vi "Handler - Set Testing State.vi"(8 "error in":errorcluster, 10 "Data In":bool, 11 "File IO Data in":T1={"Work Order Folder"=path "", "Runcount File"=path "", "Report Template Folder"=path "", "Report Folder"=path "", "Report File"=path "", "APU Setup Folder"=path "", "Testing State"=FALSE, "Recording State"=FALSE, "TDMS File Ref"=refnum, "APU Setup File Ref"=refnum, "APU Select"="<Select>", "Test Information"={"APU Part Number:"="", "Model:"="", "Serial Number:"="", "Customer:"="", "Work Order:"="", "Repair Level:"="", "Pre or Post SB"=""}, "Crash Log Data"=[], "Group Name"="", "APU Setup File"={"Sensor Info"=[], "Calibration Info"=[], "CMM Table 106"=[], "CMM Table 106B "=[], "Accel Config"=[], "Report Sheet 1"=[], "Report Sheet 2"=[], "Report Sheet 3"=[]}, "APURunCount"=0}) -> (0 "error out":errorcluster, 3 "File IO Data out":T1={"Work Order Folder"=path "", "Runcount File"=path "", "Report Template Folder"=path "", "Report Folder"=path "", "Report File"=path "", "APU Setup Folder"=path "", "Testing State"=FALSE, "Recording State"=FALSE, "TDMS File Ref"=refnum, "APU Setup File Ref"=refnum, "APU Select"="<Select>", "Test Information"={"APU Part Number:"="", "Model:"="", "Serial Number:"="", "Customer:"="", "Work Order:"="", "Repair Level:"="", "Pre or Post SB"=""}, "Crash Log Data"=[], "Group Name"="", "APU Setup File"={"Sensor Info"=[], "Calibration Info"=[], "CMM Table 106"=[], "CMM Table 106B "=[], "Accel Config"=[], "Report Sheet 1"=[], "Report Sheet 2"=[], "Report Sheet 3"=[]}, "APURunCount"=0})   [LabVIEW 2018]
doc: "Handle events that occur when the testing state changes. Includes the initialization of the TMDS file."
uses:
  Top Level/Shared Controls/Acq Data.ctl
  Top Level/Shared Controls/Calculated Data.ctl
  Top Level/Shared Controls/All Data Cluster.ctl
  Top Level/Shared Controls/Analyzed Data Sets.ctl
  Controller (Host)/Public Controls/Test Information.ctl
  Controller (Host)/Controller (Host).lvlib
  Private Controls/File IO Data.ctl
  File IO.lvlib
  Controller (Host)/Public Controls/APU Select.ctl
  Top Level/Shared Controls/APU Setup File.ctl
panel:
  # "Test Information:"
  # "Test Information:"
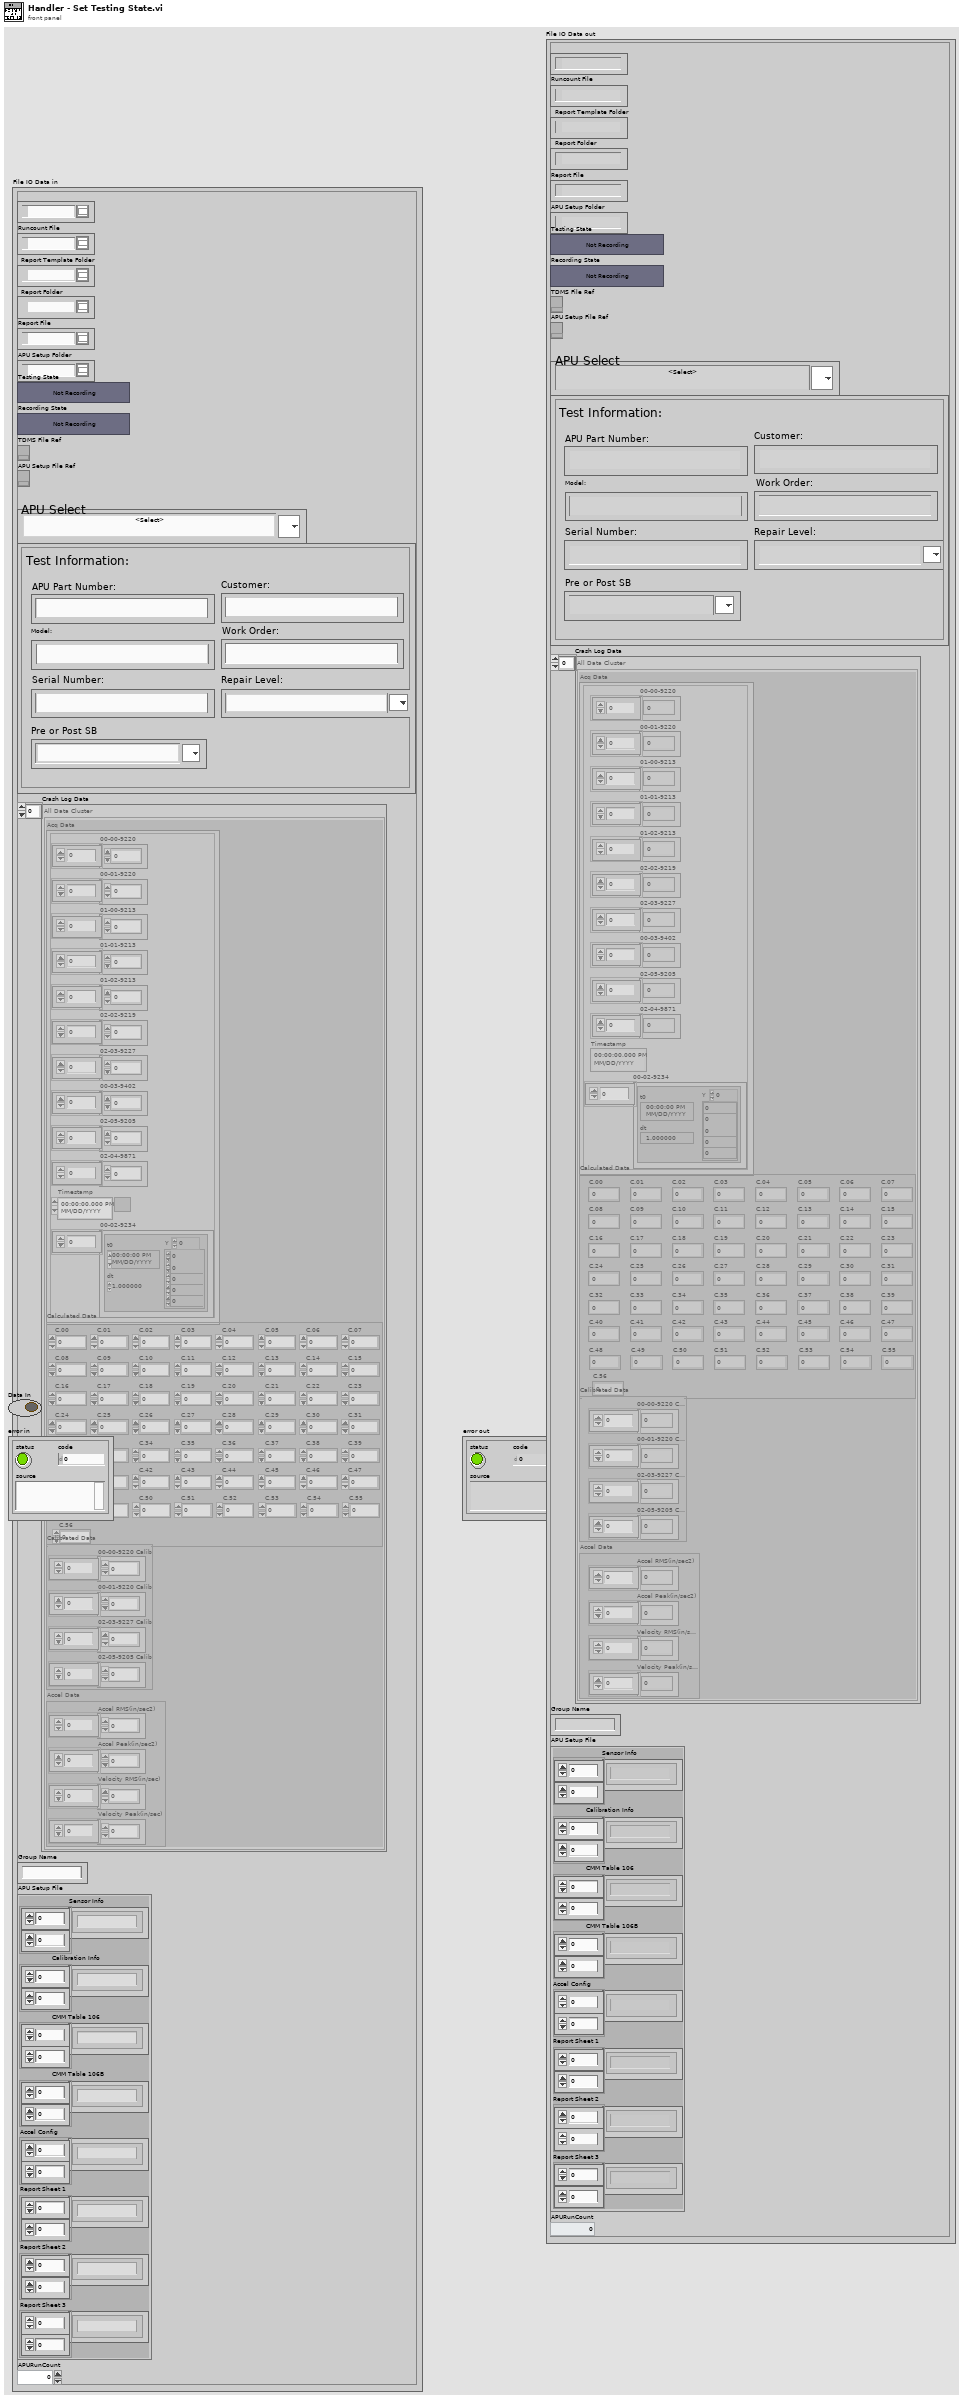
[diagram p1: front panel]
types:
  T1 = typedef "File IO.lvlib/File IO Data.ctl" = cluster{"Work Order Folder":path, "Runcount File":path, "Report Template Folder":path, "Report Folder":path, "Report File":path, "APU Setup Folder":path, "Testing State":bool, "Recording State":bool, "TDMS File Ref":refnum<k34>, "APU Setup File Ref":refnum<k34>, "APU Select":T2, "Test Information":T3, "Crash Log Data":T4, "Group Name":string, "APU Setup File":T8, "APURunCount":u32}
  T2 = typedef "Controller (Host).lvlib/APU Select.ctl" = string
  T3 = typedef "Controller (Host).lvlib/Test Information.ctl" = cluster{"APU Part Number:":string, "Model:":string, "Serial Number:":string, "Customer:":string, "Work Order:":string, "Repair Level:":string, "Pre or Post SB":string}
  T4 = typedef "Analyzed Data Sets.ctl" = T5[]
  T5 = typedef "All Data Cluster.ctl" = cluster{"Acq Data":T6, "Calculated Data":T7, "Calibrated Data":cluster{"00-00-9220 Calib":dbl[], "00-01-9220 Calib":dbl[], "02-03-9227 Calib":dbl[], "02-05-9205 Calib":dbl[]}, "Accel Data":cluster{"Accel RMS(in/sec2)":dbl[], "Accel Peak(in/sec2)":dbl[], "Velocity RMS(in/sec)":dbl[], "Velocity Peak(in/sec)":dbl[]}}
  T6 = typedef "Acq Data.ctl" = cluster{"00-00-9220":dbl[], "00-01-9220":dbl[], "01-00-9213":dbl[], "01-01-9213":dbl[], "01-02-9213":dbl[], "02-02-9219":dbl[], "02-03-9227":dbl[], "00-03-9402":dbl[], "02-05-9205":dbl[], "02-04-9871":dbl[], "Timestamp":timestamp, "00-02-9234":waveform(sgl)[]}
  T7 = typedef "Calculated Data.ctl" = cluster{"C.00":dbl, "C.01":dbl, "C.02":dbl, "C.03":dbl, "C.04":dbl, "C.05":dbl, "C.06":dbl, "C.07":dbl, "C.08":dbl, "C.09":dbl, "C.10":dbl, "C.11":dbl, "C.12":dbl, "C.13":dbl, "C.14":dbl, "C.15":dbl, "C.16":dbl, "C.17":dbl, "C.18":dbl, "C.19":dbl, "C.20":dbl, "C.21":dbl, "C.22":dbl, "C.23":dbl, "C.24":dbl, "C.25":dbl, "C.26":dbl, "C.27":dbl, "C.28":dbl, "C.29":dbl, "C.30":dbl, "C.31":dbl, "C.32":dbl, "C.33":dbl, "C.34":dbl, "C.35":dbl, "C.36":dbl, "C.37":dbl, "C.38":dbl, "C.39":dbl, "C.40":dbl, "C.41":dbl, "C.42":dbl, "C.43":dbl, "C.44":dbl, "C.45":dbl, "C.46":dbl, "C.47":dbl, "C.48":dbl, "C.49":dbl, "C.50":dbl, "C.51":dbl, "C.52":dbl, "C.53":dbl, "C.54":dbl, "C.55":dbl, "C.56":dbl}
  T8 = typedef "APU Setup File.ctl" = cluster{"Sensor Info":string[][], "Calibration Info":string[][], "CMM Table 106":string[][], "CMM Table 106B ":string[][], "Accel Config":string[][], "Report Sheet 1":string[][], "Report Sheet 2":string[][], "Report Sheet 3":string[][]}
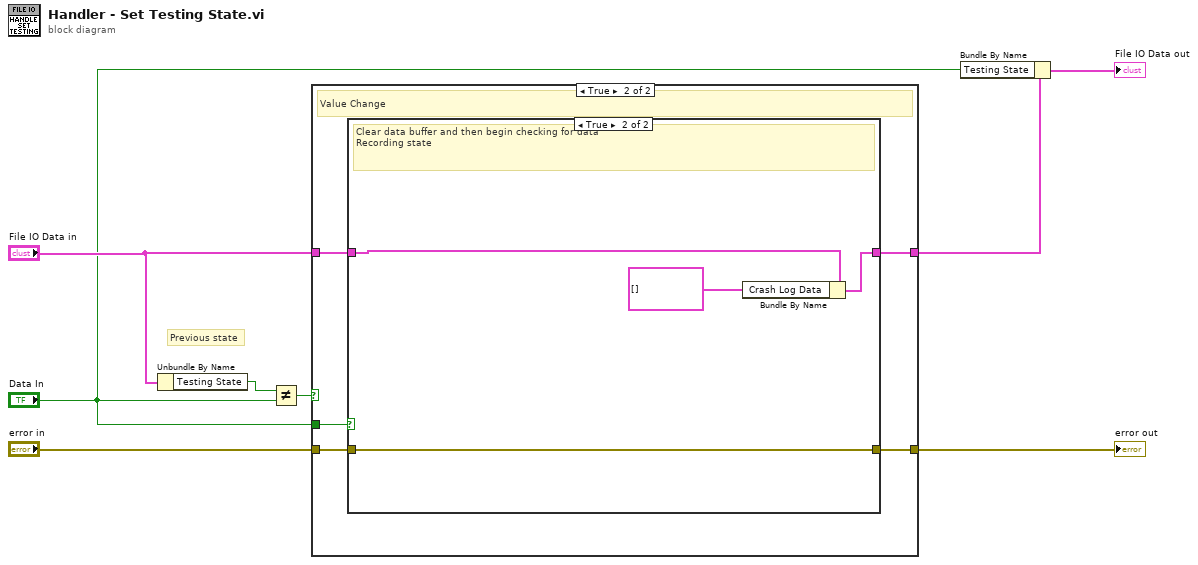
[diagram p0: block diagram]
diagram:
  # "Previous state"
  n1 = Unbundle By Name("File IO Data in") -> ("Testing State"=w2:bool)
  n2 = Not Equal?(x=w2, y="Data In") -> (x != y?=w3:bool)
  n3 = case shown="True" w3 {
    tunnel: "error in" -> [w10 w14]
    tunnel: "Data In" -> [_ w13]
    tunnel: [w10 w15] -> w6
    tunnel: "File IO Data in" -> [w9 w11]
    tunnel: [w9 w12] -> w7
    frame False {
      # "No value change, so don't do anything"
    }
    frame True {
      # "Value Change"
      n4 = case shown="True" w13 {
        tunnel: [w16 w19] -> w15
        tunnel: w14 -> [w16 w19]
        tunnel: [w17 w20] -> w12
        tunnel: w11 -> [w17 w21]
        frame False {
          # "Not recording"
        }
        frame True {
          # "Clear data buffer and then begin checking for data\nRecording state"
          n5 = Bundle By Name(cluster=w21, "Crash Log Data"=T4 []) -> (w20:T1)
        }
      }
    }
  }
  "error out" <- w6
  n6 = Bundle By Name(cluster=w7, "Testing State"="Data In") -> (→"File IO Data out":T1)
